vi "trial file path check.vi"() -> ()   [LabVIEW 2025]
panel:
  out "appended path":path
  out "FILE OUT":path
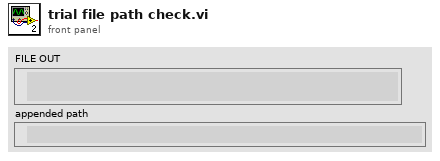
[diagram p1: front panel]
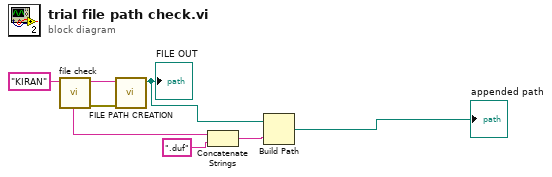
[diagram p0: block diagram]
diagram:
  w4 = "KIRAN" ("File Name In")
  n1 = call "file check.vi"("File Name In"=w4) -> ("error out"=w7:errorcluster, "File Name Out"=w6:string)  [unwired: 9 in]
  n2 = call "FILE PATH CREATION.vi"("error in"=w7, "FILE NAME :"=w6) -> ("FILE OUT"=w5:path)  [unwired: 8 in, 1 out]
  "FILE OUT" <- w5
  n3 = Concatenate Strings(w4, ".duf" ("string")) -> (w3:string)
  n4 = Build Path(base path=w5, name or relative path=w3) -> (appended path=→"appended path":path)
